vi "LPCA Interface.vi"(6 "Resistance":refnum<vi>, 7 "index":i32, 8 "error in (no error)":errorcluster, 9 "Cluster":T1={"Queue Array"=[], "Queue Element"={"state"="", "data"=variant}, "System Event"=refnum, "System Event RefNum"=refnum, "Queue List"=[], "LPCA COM"="", "Rotating"=FALSE, "PrecorAI"="", "T_0 Index"=0, "Bar Graph X"=[], "Channels"=[], "Active Indicies"=[], "Active Channels"=[], "Sample Frequency"=0.0, "Ibrake Sweep"=[], "RPM Sweep"=[], "Load Sweep"=[], "Step Height Sweep"=[], "Range Sweep"=[], "A Counter"=0, "B Counter"=0, "C Counter"=0, "#A"=0, "#B"=0, "#C"=0, "Current RPM"=0.0, "Current Ibrake"=0, "Current Range"=0, "Current Step Height"=0, "Load Bank"=enum."OFF", "Cfg Cntrls"=[], "T_Monitor Indices"=[], "Thermal Limit"=0, "Thermal Resume"=0, "Timer Reset"=FALSE, "Stop Time"=0.0, "Autotest"=FALSE, "Pulsed RPM Capture"=FALSE, "Get Sample"=FALSE, "Last State"="", "Reset Timeout"=FALSE, "Ctrl Refs"={"Test Details"=refnum, "Save Config"=refnum, "Load Config"=refnum, "Path"=refnum, "Snapshot"=refnum, "SS#"=refnum, "Ibrake"=refnum, "RPM Target"=refnum, "Spin"=refnum, "Load Bank"=refnum, "Start Test"=refnum, "Pause Test"=refnum, "Load Sweep"=refnum, "RPM Sweep"=refnum, "Ibrake Sweep"=refnum, "Filters"=refnum, "Sample Frequency"=refnum, "Data Setup"=refnum, "Pause"=refnum, "Stop Time"=refnum, "S Period"=refnum, "Range"=refnum, "Step Height"=refnum, "Step Height Sweep"=refnum, "Range Sweep"=refnum, "Available Tests"=refnum, "RPM Graph"=refnum, "RPM Knob"=refnum, "FanMode"=refnum, "Fan Mode LED Array"=refnum, "Thermal Equilibrium"=refnum, "Data Display"=refnum, "LPCA Error"=refnum, "LPCA Ramp"=refnum, "LPCA Range"=refnum, "LPCA Resistance"=refnum, "Analyze Read"=refnum, "Console Select"=refnum, "Sub Panel"=refnum}, "Pulse Waveform"={"t0"=timestamp(0 s since 1904-01-01), "dt"=1.0, "Y"=[]}, "Snapshot"={"Test Details"="test", "Version"="test", "Date"=timestamp(3493915594.3018084 s since 1904-01-01), "Selected Test"="man", "Snapshot Number"=0, "Time"=timestamp(3493915602.7292905 s since 1904-01-01), "Ibrake Setpoint"="1", "RPM Setpoint"="20", "Range Setpoint"="", "Step Height Setpoint"="", "Load Bank Setpoint"="15", "Measurement Headers"="a,b,c,1,2,3", "Measurements"="1,2,3,4,5,6,7,8", "A"=0, "B"=0, "C"=0, "Raw Data"=[], "Available Tests"=enum."Manual", "Ibrake List"="", "RPM List"="", "Load Bank List"="", "Range List"="", "Step Height List"="", "FanMode Setpoint"=enum."Auto"}, "Sample Period"=0.0, "OverTemp"=FALSE, "Available Tests"=enum."Manual", "FanMode"=enum."Auto", "Fan Mode LED Array"=[FALSE, TRUE, FALSE], "Thermal\nEquilibrium "=FALSE, "Equilibrium Stop"=FALSE, "AvgDegChg"=[]} {"Snapshot"."Time" format="%<%H:%M:%S>T"; "Snapshot"."Date" format="%<%m/%d/%Y>T"}, 10 "String":refnum<vi>) -> ()   [LabVIEW 2017]
uses:
  Controls/Test TypeDef.ctl
  Code Library/Queue References Array.ctl
  Code Library/Queue Element.ctl
  Controls/Load Bank.ctl
  Controls/Available Tests.ctl
  Console Sim/Controls/Console Select.ctl
  Controls/Snapshot Typedef.ctl
  Controls/FanMode.ctl
  Controls/LPCA Commands.ctl
  <vilib>/Instr/_visa.llb/VISA Configure Serial Port (Serial Instr).vi
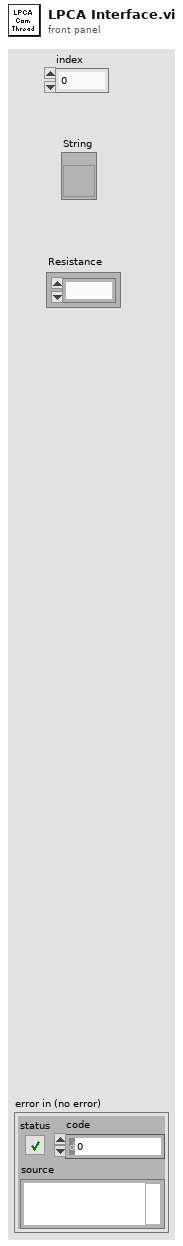
[diagram p1: front panel]
types:
  T1 = typedef "Test TypeDef.ctl" = cluster{"Queue Array":T2, "Queue Element":T3, "System Event":refnum<user-event>, "System Event RefNum":refnum<event-registration>, "Queue List":string[], "LPCA COM":refnum<visa-resource-name>, "Rotating":bool, "PrecorAI":refnum<k21>, "T_0 Index":i32, "Bar Graph X":i32[], "Channels":string[], "Active Indicies":i32[], "Active Channels":string[][], "Sample Frequency":dbl, "Ibrake Sweep":string[], "RPM Sweep":string[], "Load Sweep":string[], "Step Height Sweep":string[], "Range Sweep":string[], "A Counter":i32, "B Counter":i32, "C Counter":i32, "#A":i32, "#B":i32, "#C":i32, "Current RPM":dbl, "Current Ibrake":u32, "Current Range":u32, "Current Step Height":u32, "Load Bank":T4, "Cfg Cntrls":refnum<vi>[], "T_Monitor Indices":i32[], "Thermal Limit":i32, "Thermal Resume":i32, "Timer Reset":bool, "Stop Time":dbl, "Autotest":bool, "Pulsed RPM Capture":bool, "Get Sample":bool, "Last State":string, "Reset Timeout":bool, "Ctrl Refs":cluster{"Test Details":refnum<vi>, "Save Config":refnum<vi>, "Load Config":refnum<vi>, "Path":refnum<vi>, "Snapshot":refnum<vi>, "SS#":refnum<vi>, "Ibrake":refnum<vi>, "RPM Target":refnum<vi>, "Spin":refnum<vi>, "Load Bank":refnum<vi>, "Start Test":refnum<vi>, "Pause Test":refnum<vi>, "Load Sweep":refnum<vi>, "RPM Sweep":refnum<vi>, "Ibrake Sweep":refnum<vi>, "Filters":refnum<vi>, "Sample Frequency":refnum<vi>, "Data Setup":refnum<vi>, "Pause":refnum<vi>, "Stop Time":refnum<vi>, "S Period":refnum<vi>, "Range":refnum<vi>, "Step Height":refnum<vi>, "Step Height Sweep":refnum<vi>, "Range Sweep":refnum<vi>, "Available Tests":refnum<vi>, "RPM Graph":refnum<vi>, "RPM Knob":refnum<vi>, "FanMode":refnum<vi>, "Fan Mode LED Array":refnum<vi>, "Thermal Equilibrium":refnum<vi>, "Data Display":refnum<vi>, "LPCA Error":refnum<vi>, "LPCA Ramp":refnum<vi>, "LPCA Range":refnum<vi>, "LPCA Resistance":refnum<vi>, "Analyze Read":refnum<vi>, "Console Select":refnum<vi>, "Sub Panel":refnum<vi>}, "Pulse Waveform":waveform(dbl), "Snapshot":T5, "Sample Period":dbl, "OverTemp":bool, "Available Tests":T6, "FanMode":T7, "Fan Mode LED Array":bool[], "Thermal\nEquilibrium ":bool, "Equilibrium Stop":bool, "AvgDegChg":dbl[]}
  T2 = typedef "Queue References Array.ctl" = refnum<queue>[]
  T3 = typedef "Queue Element.ctl" = cluster{"state":string, "data":variant}
  T4 = typedef "Load Bank.ctl" = enum16{"OFF", "50", "25", "16.7", "12.5", "10.0", "8.3", "7.1", "6.3", "5.6", "5.0", "4.5", "4.2", "3.8", "3.6", "3.3", "3.1"}
  T5 = typedef "Snapshot Typedef.ctl" = cluster{"Test Details":string, "Version":string, "Date":timestamp, "Selected Test":string, "Snapshot Number":u16, "Time":timestamp, "Ibrake Setpoint":string, "RPM Setpoint":string, "Range Setpoint":string, "Step Height Setpoint":string, "Load Bank Setpoint":string, "Measurement Headers":string, "Measurements":string, "A":i32, "B":i32, "C":i32, "Raw Data":string[][], "Available Tests":T6, "Ibrake List":string, "RPM List":string, "Load Bank List":string, "Range List":string, "Step Height List":string, "FanMode Setpoint":T7}
  T6 = typedef "Available Tests.ctl" = enum16{"Manual", "EFX Brake Torque", "Generator Torque", "EFX Brake Thermal", "Generator Thermal", "Pulsed RPM", "AMT Brake Torque", "Bike Brake Torque", "AMT Brake Thermal", "Bike Brake Thermal"}
  T7 = typedef "FanMode.ctl" = enum16{"On", "Off", "Auto"}
  T8 = typedef "LPCA Commands.ctl" = enum16{"RSET", "stop", "rpmh", "rpml", "prpm", "rpm", "mamp", "rng", "tmp1", "tmp2", "err", "ramp"}
  T9 = enum16{"Init", "Get", "Set Step Counter", "Insert Command", "Insert Now Command"}
  T10 = cluster{"Test Details":refnum<vi>, "Save Config":refnum<vi>, "Load Config":refnum<vi>, "Path":refnum<vi>, "Snapshot":refnum<vi>, "SS#":refnum<vi>, "Ibrake":refnum<vi>, "RPM Target":refnum<vi>, "Spin":refnum<vi>, "Load Bank":refnum<vi>, "Start Test":refnum<vi>, "Pause Test":refnum<vi>, "Load Sweep":refnum<vi>, "RPM Sweep":refnum<vi>, "Ibrake Sweep":refnum<vi>, "Filters":refnum<vi>, "Sample Frequency":refnum<vi>, "Data Setup":refnum<vi>, "Pause":refnum<vi>, "Stop Time":refnum<vi>, "S Period":refnum<vi>, "Range":refnum<vi>, "Step Height":refnum<vi>, "Step Height Sweep":refnum<vi>, "Range Sweep":refnum<vi>, "Available Tests":refnum<vi>, "RPM Graph":refnum<vi>, "RPM Knob":refnum<vi>, "FanMode":refnum<vi>, "Fan Mode LED Array":refnum<vi>, "Thermal Equilibrium":refnum<vi>, "Data Display":refnum<vi>, "LPCA Error":refnum<vi>, "LPCA Ramp":refnum<vi>, "LPCA Range":refnum<vi>, "LPCA Resistance":refnum<vi>, "Analyze Read":refnum<vi>, "Console Select":refnum<vi>, "Sub Panel":refnum<vi>}
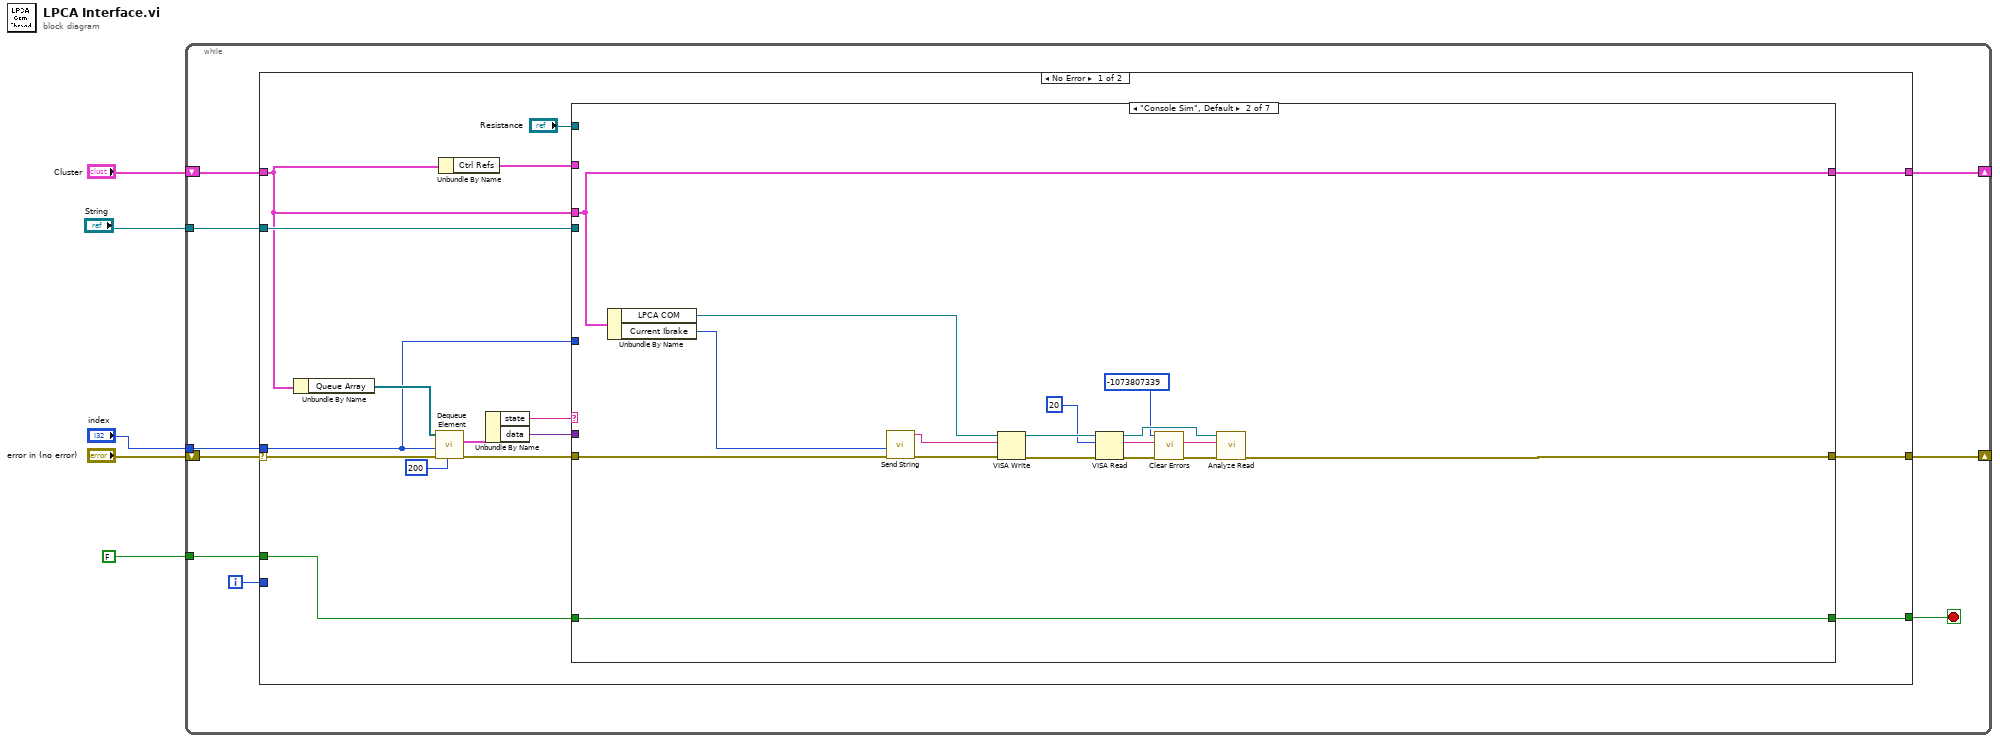
[diagram p0: block diagram]
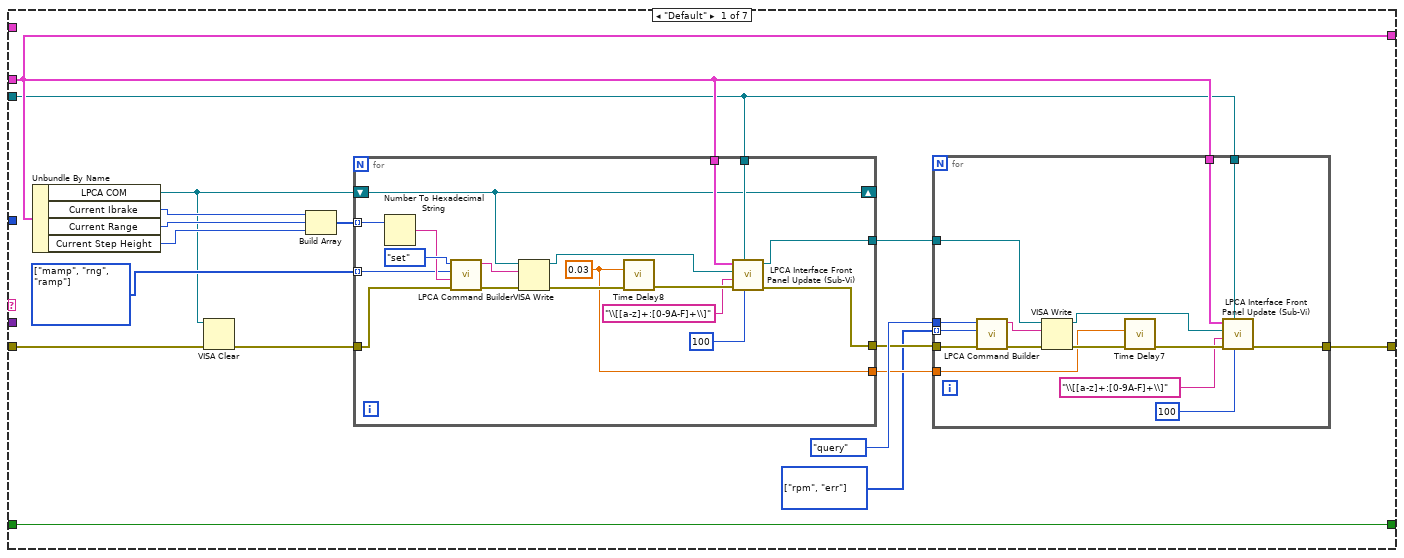
[diagram p2: hidden frame]
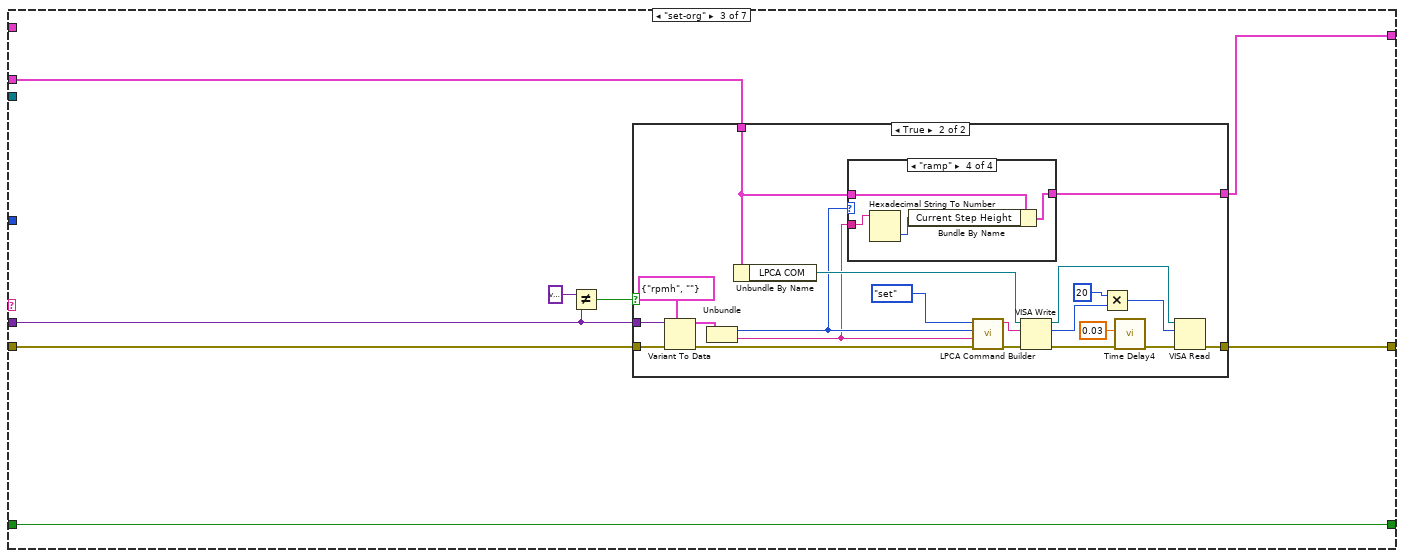
[diagram p3: hidden frame]
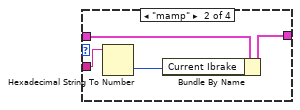
[diagram p6: hidden frame]
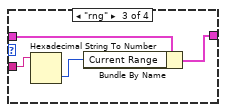
[diagram p7: hidden frame]
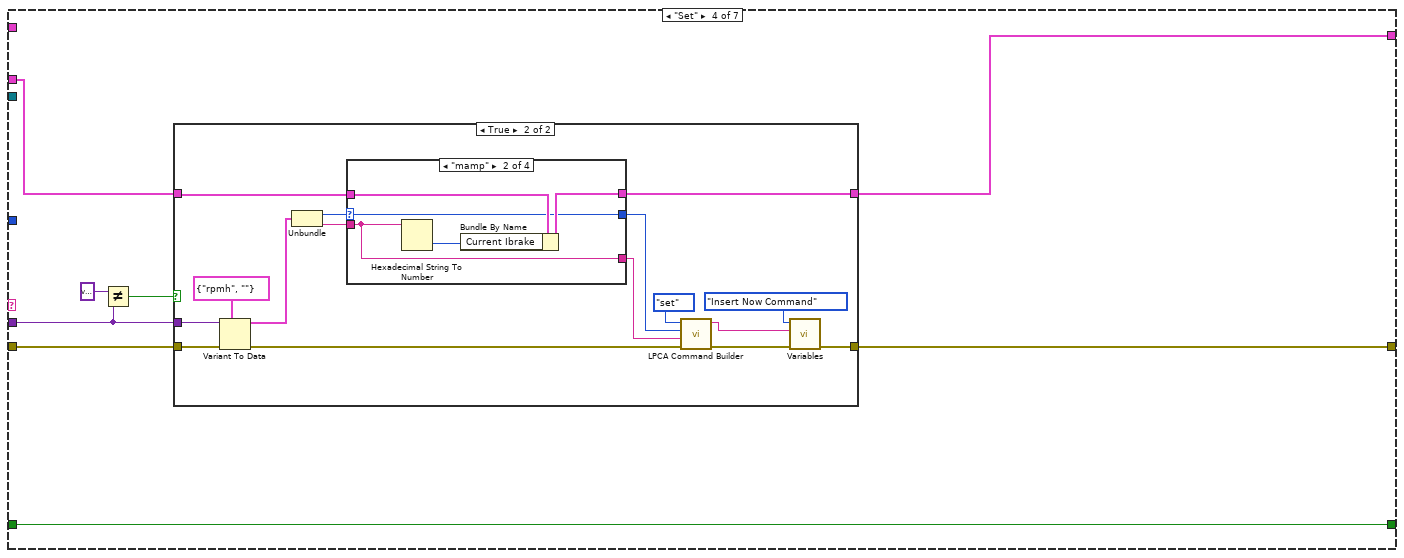
[diagram p8: hidden frame]
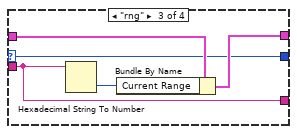
[diagram p11: hidden frame]
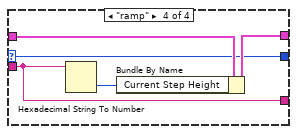
[diagram p12: hidden frame]
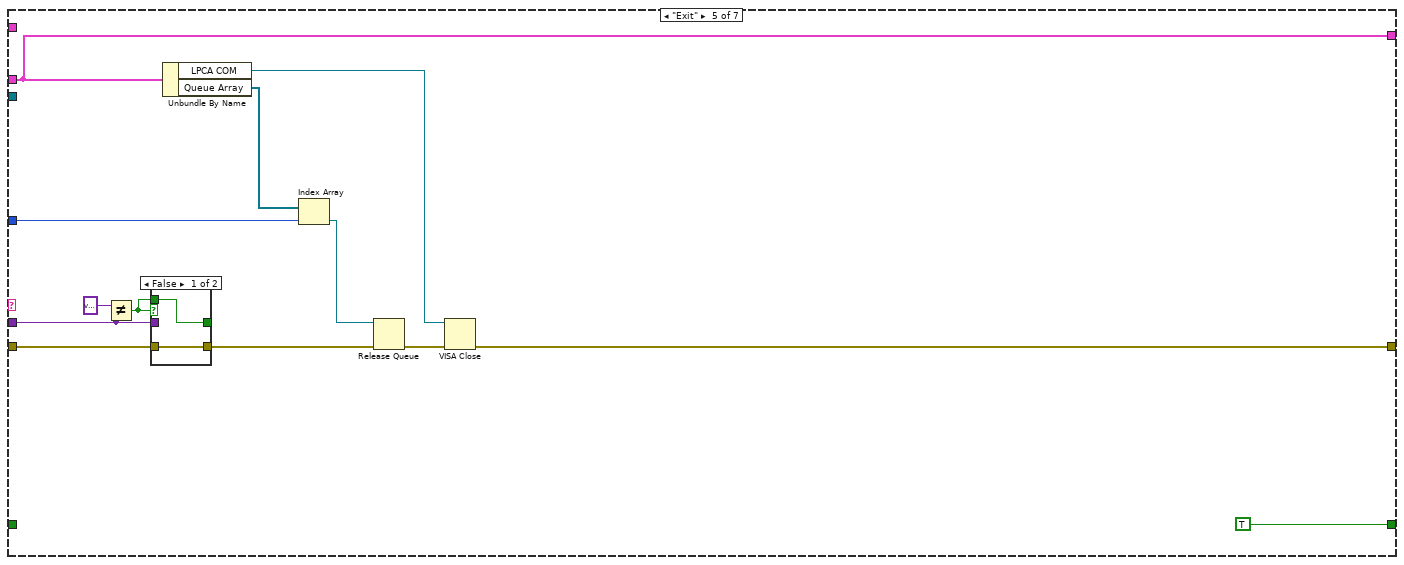
[diagram p13: hidden frame]
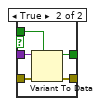
[diagram p14: hidden frame]
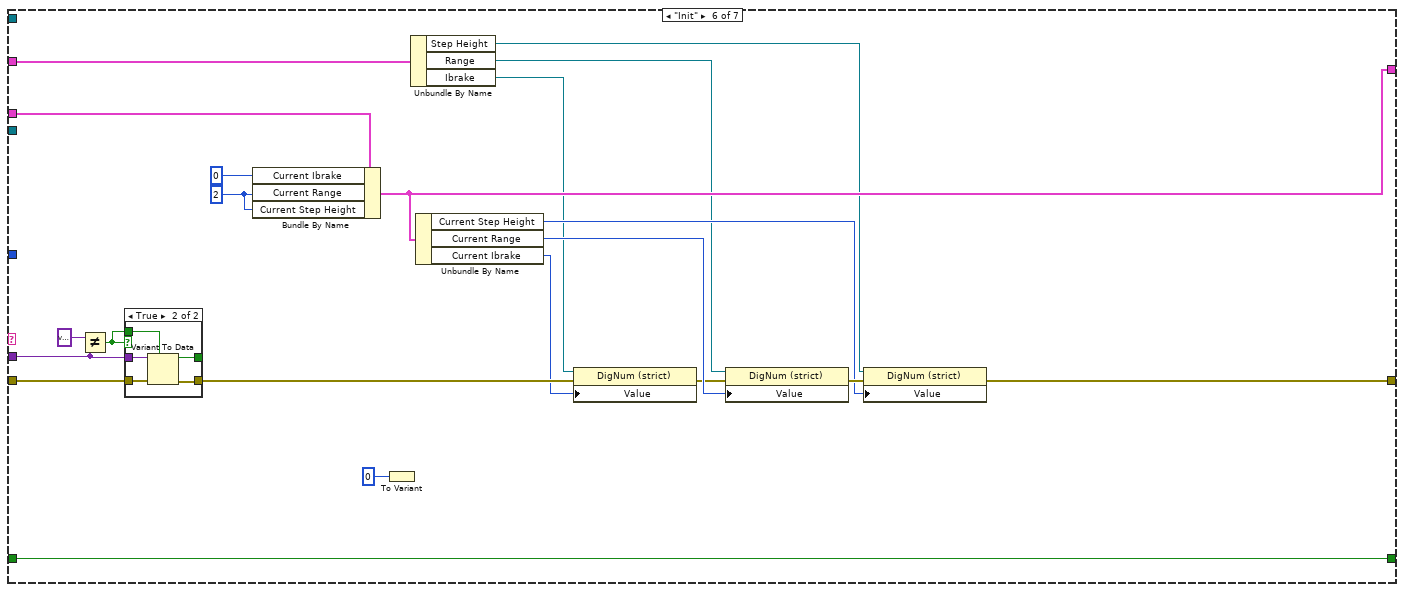
[diagram p15: hidden frame]
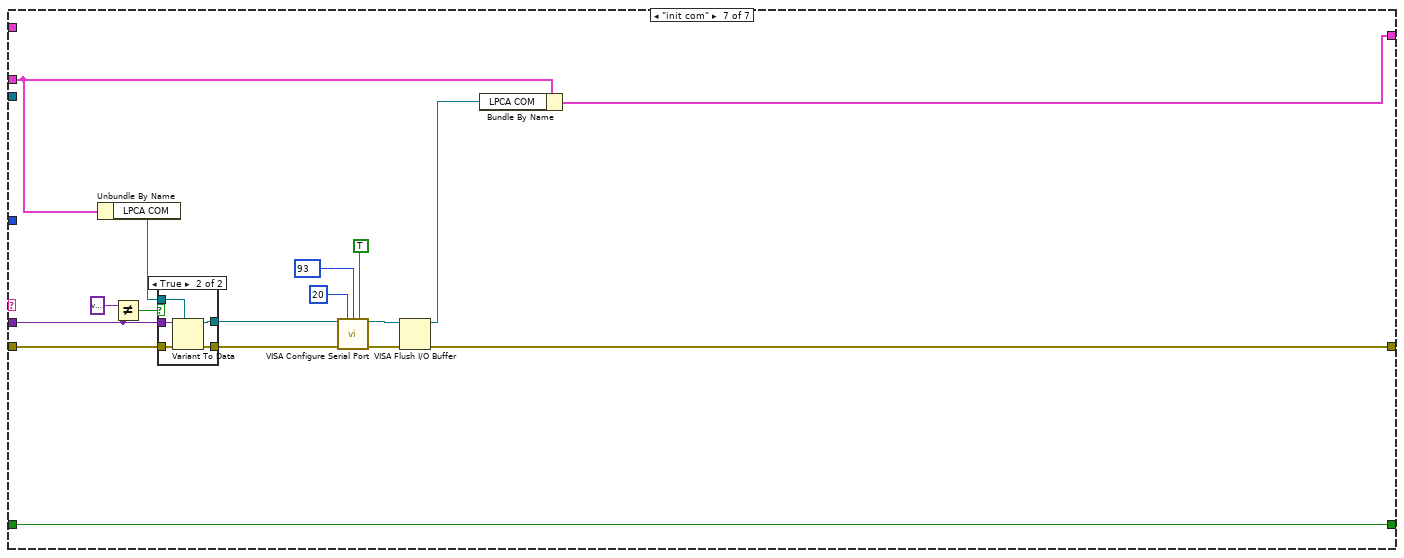
[diagram p17: hidden frame]
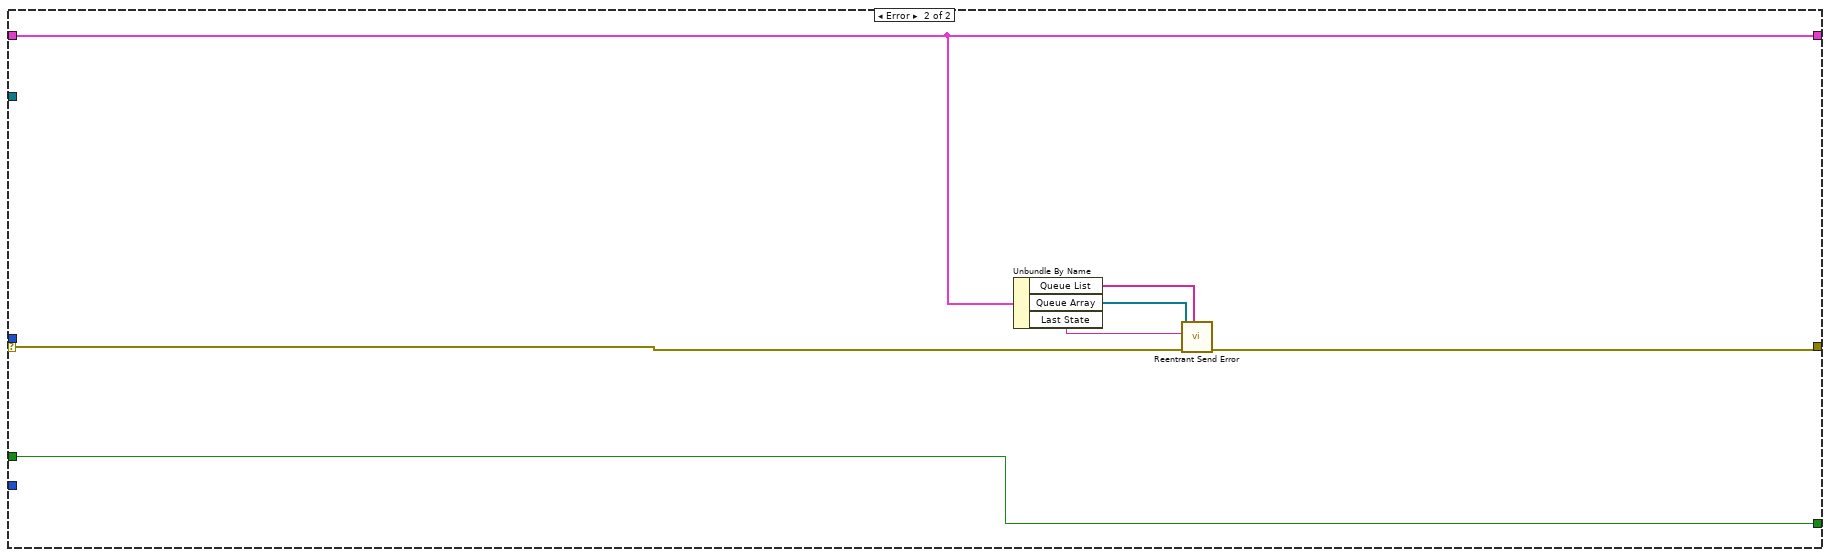
[diagram p19: hidden frame]
diagram:
  n1 = while {
    shift-right: [w9] -> _
    shift-left: "Cluster" -> [w14]
    tunnel: FALSE ("Boolean") -> [w11]
    shift-right: [w12] -> _
    shift-left: "error in (no error)" -> [w13]
    tunnel: "index" -> [w8]
    tunnel: "String" -> [w7]
    i -> [w6]
    stop <- w10 stop-if-true
    n2 = case shown="No Error" w13 {
      selector: w13 -> [w28 w259]
      tunnel: w14 -> [w15 w257]
      tunnel: [w26 w258] -> w12
      tunnel: w11 -> [w25 w263]
      tunnel: [w24 w263] -> w10
      tunnel: [w21 w257] -> w9
      tunnel: w8 -> [w17 _]
      tunnel: w7 -> [w20 _]
      tunnel: w6 -> [_ _]
      frame No Error {
        n3 = Unbundle By Name(w15) -> ("Queue Array"=w30:T2)
        n4 = call "Dequeue Element.vi"("timeout in ms (-1)"=200, "error in (no error)"=w28, "index"=w17, "Queue Array"=w30) -> ("error out"=w27:errorcluster, "Queue Element"=w19:T3)  [unwired: 5 in, 1 out]
        n5 = Unbundle By Name(w15) -> ("Ctrl Refs"=w16:T10)
        n6 = Unbundle By Name(w19) -> ("state"=w23:string, "data"=w22:variant)
        n7 = case shown="\"Console Sim\", Default" w23 {
          tunnel: w27 -> [w33 w91 w103 w147 w197 w224 w248]
          tunnel: [w36 w85 w100 w144 w190 w205 w236] -> w26
          tunnel: w25 -> [w47 w96 w104 w148 _ w225 w249]
          tunnel: [w47 w96 w104 w148 TRUE ("Boolean") w225 w249] -> w24
          tunnel: w22 -> [_ _ w101 w145 w195 w222 w246]
          tunnel: [w35 w95 w97 w141 w193 w213 w244] -> w21
          tunnel: w15 -> [w35 w95 w98 w142 w193 w216 w243]
          tunnel: w20 -> [w34 _ _ _ _ _ _]
          tunnel: "Resistance" -> [_ _ _ _ _ _ _]
          tunnel: w17 -> [_ _ _ _ w187 _ _]
          tunnel: w16 -> [_ _ _ _ _ w212 _]
          frame "Default" {
            w37 = T8[] [enum."rpm", enum."err"] items=["RSET", "stop", "rpmh", "rpml", "prpm", "rpm", "mamp", "rng", "tmp1", "tmp2", "err", "ramp"]
            w41 = T8[] [enum."mamp", enum."rng", enum."ramp"] items=["RSET", "stop", "rpmh", "rpml", "prpm", "rpm", "mamp", "rng", "tmp1", "tmp2", "err", "ramp"]
            n8 = Unbundle By Name(w35) -> ("LPCA COM"=w31:refnum<visa-resource-name>, "Current Ibrake"=w45:u32, "Current Range"=w44:u32, "Current Step Height"=w43:u32)
            n9 = VISA Clear(VISA resource name=w31, error in (no error)=w33) -> (error out=w32:errorcluster)  [unwired: 1 out]
            n10 = Build Array(w45, w44, w43) -> (w42:u32[])
            n11 = for {
              tunnel: w42 -> [w60] mode=indexing
              tunnel: w41 -> [w59] mode=indexing
              tunnel: [w50] -> w40
              tunnel: w32 -> [w58]
              tunnel: [w56] -> w39
              tunnel: [w57] -> w38
              tunnel: w34 -> [w55]
              tunnel: w35 -> [w54]
              shift-right: [w48] -> _
              shift-left: w31 -> [w48]
              w57 = 0.03 ("Delay Time (s)")
              n12 = Number To Hexadecimal String(2:w60) -> (0:w62:string)  [unwired: 1 in]
              n13 = call "LPCA Command Builder.vi"("error in (no error)"=w58, "Data"=w62, "LPCA Command"=w59, "Mode"=enum16{"set", "query"}."set") -> ("error out"=w63:errorcluster, "String"=w64:string)  [unwired: 6 in]
              n14 = VISA Write(VISA resource name=w48, write buffer=w64, error in (no error)=w63) -> (VISA resource name out=w52:refnum<visa-resource-name>, error out=w61:errorcluster)  [unwired: 1 out]
              n15 = call "Time Delay8"("error in (no error)"=w61, "Delay Time (s)"=w57) -> ("error out"=w53:errorcluster)  [unwired: 9 in]
              n16 = call "LPCA Interface Front Panel Update (Sub-Vi).vi"("byte count"=u32 100, "String"=w55, "error in (no error)"=w53, "regular expression"="\\[[a-z]+:[0-9A-F]+\\]", "VISA resource name"=w52, "Cluster"=w54) -> ("error out"=w56:errorcluster, "VISA resource out"=w50:refnum<visa-resource-name>)  [unwired: 4 in]
            }
            n17 = for {
              tunnel: enum16{"set", "query"}."query" ("Mode") -> [w79]
              tunnel: w39 -> [w78]
              tunnel: w40 -> [w77]
              tunnel: w37 -> [w76] mode=indexing
              tunnel: w38 -> [w74]
              tunnel: [w67] -> w36
              tunnel: w35 -> [w71]
              tunnel: w34 -> [w70]
              n18 = call "LPCA Command Builder.vi"("error in (no error)"=w78, "LPCA Command"=w76, "Mode"=w79) -> ("error out"=w80:errorcluster, "String"=w66:string)  [unwired: 7 in]
              n19 = VISA Write(VISA resource name=w77, write buffer=w66, error in (no error)=w80) -> (VISA resource name out=w72:refnum<visa-resource-name>, error out=w75:errorcluster)  [unwired: 1 out]
              n20 = call "Time Delay7"("error in (no error)"=w75, "Delay Time (s)"=w74) -> ("error out"=w73:errorcluster)  [unwired: 9 in]
              n21 = call "LPCA Interface Front Panel Update (Sub-Vi).vi"("byte count"=u32 100, "String"=w70, "error in (no error)"=w73, "regular expression"="\\[[a-z]+:[0-9A-F]+\\]", "VISA resource name"=w72, "Cluster"=w71) -> ("error out"=w67:errorcluster)  [unwired: 4 in, 1 out]
            }
          }
          frame "Console Sim", Default {
            n22 = Unbundle By Name(w95) -> ("LPCA COM"=w88:refnum<visa-resource-name>, "Current Ibrake"=w81:u32)
            n23 = call "Send String.vi"("error in (no error)"=w91, "MAMP2"=w81) -> ("error out"=w90:errorcluster, "Message"=w84:string)  [unwired: 8 in]
            n24 = VISA Write(VISA resource name=w88, write buffer=w84, error in (no error)=w90) -> (VISA resource name out=w94:refnum<visa-resource-name>, error out=w93:errorcluster)  [unwired: 1 out]
            n25 = VISA Read(VISA resource name=w94, byte count=u32 20, error in (no error)=w93) -> (VISA resource name out=w86:refnum<visa-resource-name>, read buffer=w87:string, error out=w89:errorcluster)  [unwired: 1 out]
            n26 = call <vilib>:"Clear Errors.vi"("error in (no error)"=w89, "specific error code to clear (0: all)"=-1073807339) -> ("error out"=w83:errorcluster)  [unwired: 4 in, 1 out]
            n27 = call "Analyze Read.vi"("VISA in"=w86, "String"=w87, "error in (no error)"=w83) -> ("error out"=w85:errorcluster)  [unwired: 5 in, 2 out]
          }
          frame "set-org" {
            n28 = Not Equal?(x=variant, y=w101) -> (x != y?=w99:bool)
            n29 = case shown="True" w99 {
              tunnel: w103 -> [w106 w127]
              tunnel: w101 -> [_ w126]
              tunnel: w98 -> [w105 w117]
              tunnel: [w106 w110] -> w100
              tunnel: [w105 w115] -> w97
              frame False {
              }
              frame True {
                n30 = Variant To Data(error in=w127, type=cluster{T8, string} {enum."rpmh", ""}, Variant=w126) -> (data=w119:cluster{T8, string}, error out=w124:errorcluster)
                n31 = Unbundle(w119) -> (w118:T8, w116:string)
                n32 = Unbundle By Name(w117) -> ("LPCA COM"=w125:refnum<visa-resource-name>)
                n33 = case shown="\"ramp\"" w118 {
                  tunnel: w117 -> [w128 w132 w136 w140]
                  tunnel: w116 -> [_ w130 w134 w138]
                  tunnel: [w128 w131 w135 w139] -> w115
                  frame "RSET", Default {
                  }
                  frame "mamp" {
                    n34 = Hexadecimal String To Number(string=w130) -> (number=w129:u32)  [unwired: 2 in, 1 out]
                    n35 = Bundle By Name(cluster=w132, "Current Ibrake"=w129) -> (w131:T1)
                  }
                  frame "rng" {
                    n36 = Hexadecimal String To Number(string=w134) -> (number=w133:u32)  [unwired: 2 in, 1 out]
                    n37 = Bundle By Name(cluster=w136, "Current Range"=w133) -> (w135:T1)
                  }
                  frame "ramp" {
                    n38 = Hexadecimal String To Number(string=w138) -> (number=w137:u32)  [unwired: 2 in, 1 out]
                    n39 = Bundle By Name(cluster=w140, "Current Step Height"=w137) -> (w139:T1)
                  }
                }
                n40 = call "LPCA Command Builder.vi"("error in (no error)"=w124, "Data"=w116, "LPCA Command"=w118, "Mode"=enum16{"set", "query"}."set") -> ("error out"=w121:errorcluster, "String"=w122:string)  [unwired: 6 in]
                n41 = VISA Write(VISA resource name=w125, write buffer=w122, error in (no error)=w121) -> (VISA resource name out=w109:refnum<visa-resource-name>, return count=w108:u32, error out=w111:errorcluster)
                n42 = Multiply(x=u32 20 ("byte count"), y=w108) -> (x*y=w114:u32)
                n43 = call "Time Delay4"("error in (no error)"=w111, "Delay Time (s)"=0.03) -> ("error out"=w113:errorcluster)  [unwired: 9 in]
                n44 = VISA Read(VISA resource name=w109, byte count=w114, error in (no error)=w113) -> (error out=w110:errorcluster)  [unwired: 3 out]
              }
            }
          }
          frame "Set" {
            n45 = Not Equal?(x=variant, y=w145) -> (x != y?=w143:bool)
            n46 = case shown="True" w143 {
              tunnel: w147 -> [w150 w166]
              tunnel: w145 -> [_ w165]
              tunnel: w142 -> [w149 w162]
              tunnel: [w150 w153] -> w144
              tunnel: [w149 w160] -> w141
              frame False {
              }
              frame True {
                n47 = Variant To Data(error in=w166, type=cluster{T8, string} {enum."rpmh", ""}, Variant=w165) -> (data=w152:cluster{T8, string}, error out=w156:errorcluster)
                n48 = Unbundle(w152) -> (w163:T8, w161:string)
                n49 = case shown="\"mamp\"" w163 {
                  selector: w163 -> [w168 w171 w176 w181]
                  tunnel: w162 -> [w169 w174 w179 w184]
                  tunnel: w161 -> [w167 w170 w175 w180]
                  tunnel: [w169 w173 w178 w183] -> w160
                  tunnel: [w168 w171 w176 w181] -> w158
                  tunnel: [w167 w170 w175 w180] -> w157
                  frame "RSET", Default {
                  }
                  frame "mamp" {
                    n50 = Hexadecimal String To Number(string=w170) -> (number=w172:u32)  [unwired: 2 in, 1 out]
                    n51 = Bundle By Name(cluster=w174, "Current Ibrake"=w172) -> (w173:T1)
                  }
                  frame "rng" {
                    n52 = Hexadecimal String To Number(string=w175) -> (number=w177:u32)  [unwired: 2 in, 1 out]
                    n53 = Bundle By Name(cluster=w179, "Current Range"=w177) -> (w178:T1)
                  }
                  frame "ramp" {
                    n54 = Hexadecimal String To Number(string=w180) -> (number=w182:u32)  [unwired: 2 in, 1 out]
                    n55 = Bundle By Name(cluster=w184, "Current Step Height"=w182) -> (w183:T1)
                  }
                }
                n56 = call "LPCA Command Builder.vi"("error in (no error)"=w156, "Data"=w157, "LPCA Command"=w158, "Mode"=enum16{"set", "query"}."set") -> ("error out"=w155:errorcluster, "String"=w154:string)  [unwired: 6 in]
                n57 = call "Variables.vi"("error in (no error)"=w155, "Value"=w154, "Command"=T9."Insert Now Command") -> ("error out"=w153:errorcluster)  [unwired: 6 in, 2 out]
              }
            }
          }
          frame "Exit" {
            n58 = Not Equal?(x=variant, y=w195) -> (x != y?=w194:bool)
            n59 = case shown="False" w194 {
              tunnel: w197 -> [w199 w204]
              tunnel: [w199 w203] -> w192
              tunnel: w195 -> [_ w202]
              tunnel: [w198 w201] -> _
              tunnel: w194 -> [w198 w200]
              frame False {
              }
              frame True {
                n60 = Variant To Data(error in=w204, type=w200, Variant=w202) -> (data=w201:bool, error out=w203:errorcluster)
              }
            }
            n61 = Unbundle By Name(w193) -> ("LPCA COM"=w189:refnum<visa-resource-name>, "Queue Array"=w188:T2)
            n62 = Index Array(array=w188, index=w187) -> (element=w186:refnum<queue>)
            n63 = Release Queue(queue=w186, error in (no error)=w192) -> (error out=w191:errorcluster)  [unwired: 1 in, 2 out]
            n64 = VISA Close(VISA resource name=w189, error in (no error)=w191) -> (error out=w190:errorcluster)
          }
          frame "Init" {
            w219 = u32 2 ("Resistance Range")
            n65 = Not Equal?(x=variant, y=w222) -> (x != y?=w221:bool)
            n66 = case shown="True" w221 {
              tunnel: w224 -> [w227 w232]
              tunnel: [w227 w231] -> w208
              tunnel: w222 -> [_ w230]
              tunnel: [w226 w229] -> _
              tunnel: w221 -> [w226 w228]
              frame False {
              }
              frame True {
                n67 = Variant To Data(error in=w232, type=w228, Variant=w230) -> (data=w229:bool, error out=w231:errorcluster)
              }
            }
            n68 = Bundle By Name(cluster=w216, "Current Ibrake"=u32 0 ("Current Resistance"), "Current Range"=w219, "Current Step Height"=w219) -> (w213:T1)
            n69 = To Variant(anything=u32 0 ("Resistance Range")) -> ()  [unwired: 1 out]
            n70 = Unbundle By Name(w212) -> ("Step Height"=w210:refnum<vi>, "Range"=w211:refnum<vi>, "Ibrake"=w206:refnum<vi>)
            n71 = Unbundle By Name(w213) -> ("Current Step Height"=w215:u32, "Current Range"=w214:u32, "Current Ibrake"=w207:u32)
            n72 = property class="DigNum (strict)"(reference=w206, error in=w208, "Value"=w207) -> (error out=w209:errorcluster)  [unwired: 1 out]
            n73 = property class="DigNum (strict)"(reference=w211, error in=w209, "Value"=w214) -> (error out=w217:errorcluster)  [unwired: 1 out]
            n74 = property class="DigNum (strict)"(reference=w210, error in=w217, "Value"=w215) -> (error out=w205:errorcluster)  [unwired: 1 out]
          }
          frame "init com" {
            n75 = Unbundle By Name(w243) -> ("LPCA COM"=w233:refnum<visa-resource-name>)
            n76 = Not Equal?(x=variant, y=w246) -> (x != y?=w245:bool)
            n77 = case shown="True" w245 {
              tunnel: w248 -> [w251 w256]
              tunnel: [w251 w255] -> w237
              tunnel: w246 -> [_ w254]
              tunnel: [w250 w253] -> w234
              tunnel: w233 -> [w250 w252]
              frame False {
              }
              frame True {
                n78 = Variant To Data(error in=w256, type=w252, Variant=w254) -> (data=w253:refnum<visa-resource-name>, error out=w255:errorcluster)
              }
            }
            n79 = call-poly "VISA Configure Serial Port"("VISA resource name"=w234, "timeout (10sec)"=u32 20, "termination char\n(0xA = '\\n' = LF)"=u8 93 ("termination char\n(0xA = '\\n' = LF)"), "Enable Termination\nChar (T)"=TRUE ("Enable Termination\nChar (T)"), "error in (no error)"=w237) -> ("VISA resource name out"=w240:refnum<visa-resource-name>, "error out"=w239:errorcluster)  [unwired: 9 in]
            n80 = VISA Flush I/O Buffer(VISA resource name=w240, error in (no error)=w239) -> (VISA resource name out=w235:refnum<visa-resource-name>, error out=w236:errorcluster)  [unwired: 1 in]
            n81 = Bundle By Name(cluster=w243, "LPCA COM"=w235) -> (w244:T1)
          }
        }
      }
      frame Error {
        n82 = Unbundle By Name(w257) -> ("Queue List"=w260:string[], "Queue Array"=w261:T2, "Last State"=w262:string)
        n83 = call "Reentrant Send Error.vi"("Queue Names"=w260, "error in (no error)"=w259, "Last State"=w262, "Queues"=w261) -> ("error out"=w258:errorcluster)  [unwired: 7 in]
      }
    }
  }
